vi "Acceleration.vi"() -> ()   [LabVIEW 2021]
uses:
  <vilib>/Instr/_visa.llb/VISA Configure Serial Port (Instr).vi
panel:
  out "AccelZ Chart":dbl(graph)
  out "AccelZ":dbl
  out "AccelY Chart":dbl(graph)
  out "AccelY":dbl
  out "AccelX Chart":dbl(graph)
  out "AccelX":dbl
  in  "stop":bool
  out "read buffer":string
  in  "baud rate (9600)":u32=9600
  in  "VISA resource name":refnum<visa-resource-name>
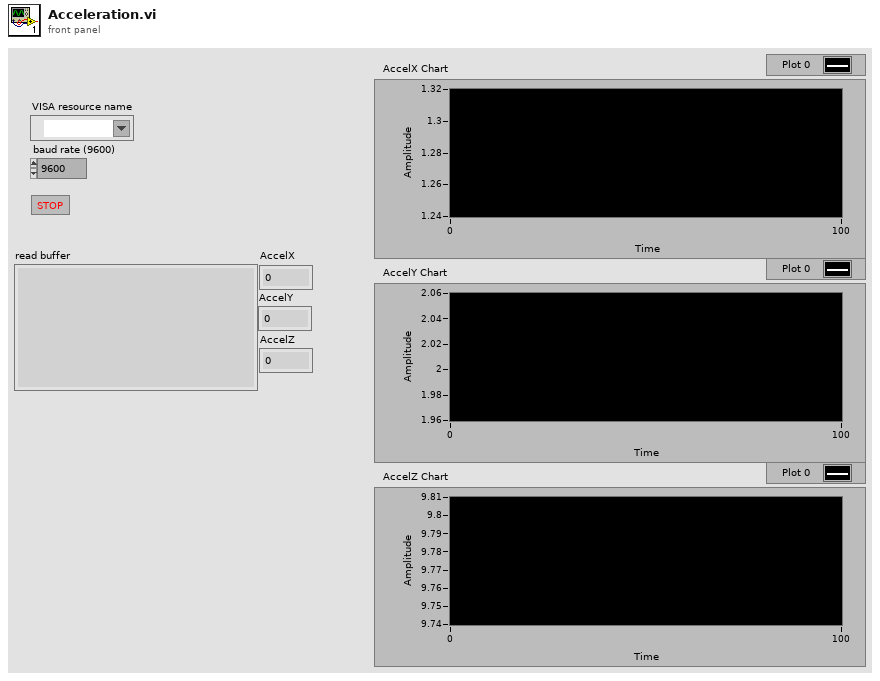
[diagram p1: front panel]
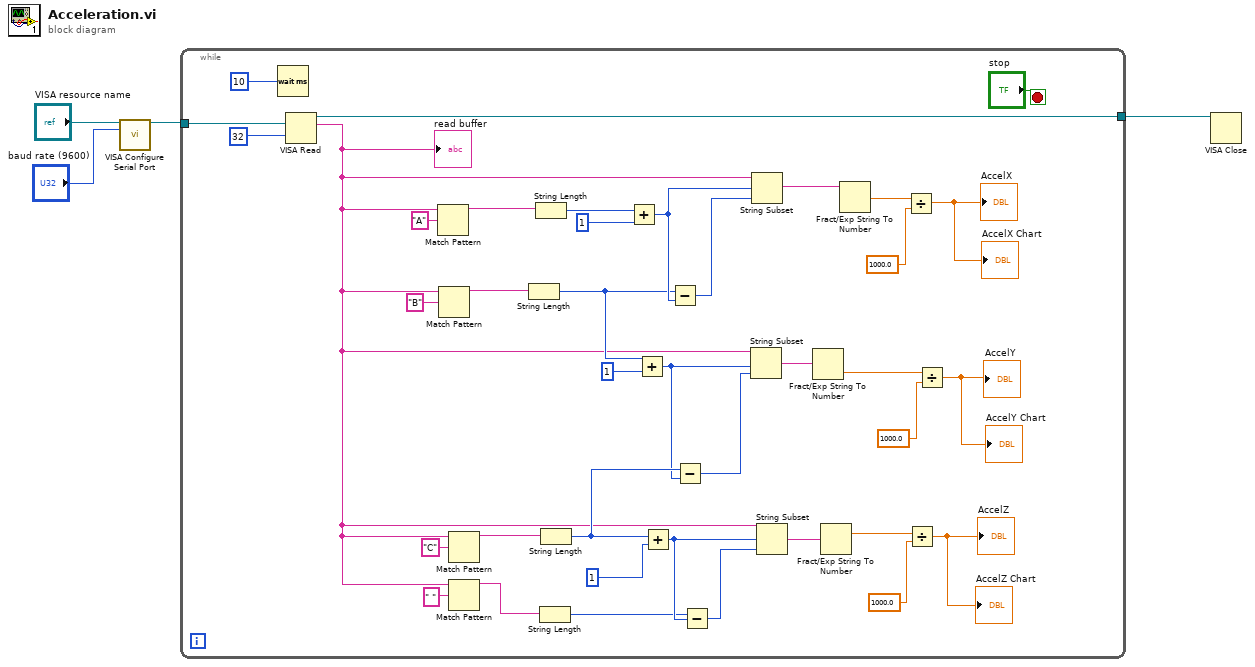
[diagram p0: block diagram]
diagram:
  n1 = call-poly "VISA Configure Serial Port"("VISA resource name"="VISA resource name", "baud rate (9600)"="baud rate (9600)") -> ("VISA resource name out"=w2:refnum<visa-resource-name>)  [unwired: 12 in, 1 out]
  n2 = while {
    tunnel: w2 -> [w43]
    tunnel: [w40] -> w1
    stop <- "stop" stop-if-true
    n3 = Wait (ms)(milliseconds to wait=u32 10) -> ()  [unwired: 1 out]
    n4 = VISA Read(VISA resource name=w43, byte count=u32 32) -> (VISA resource name out=w40:refnum<visa-resource-name>, read buffer=w15:string)  [unwired: 1 in, 2 out]
    "read buffer" <- w15
    n5 = Match Pattern(string=w15, regular expression="A") -> (before substring=w24:string)  [unwired: 1 in, 3 out]
    n6 = Match Pattern(string=w15, regular expression="B") -> (before substring=w34:string)  [unwired: 1 in, 3 out]
    n7 = Match Pattern(string=w15, regular expression="C") -> (before substring=w31:string)  [unwired: 1 in, 3 out]
    n8 = Match Pattern(string=w15, regular expression=" ") -> (before substring=w20:string)  [unwired: 1 in, 3 out]
    n9 = String Length(string=w34) -> (length=w27:i32)
    n10 = String Length(string=w24) -> (length=w36:i32)
    n11 = String Length(string=w20) -> (length=w14:i32)
    n12 = String Length(string=w31) -> (length=w26:i32)
    n13 = Add(x=w36, y=1) -> (x+y=w33:i32)
    n14 = Add(x=w27, y=1) -> (x+y=w25:i32)
    n15 = Add(x=w26, y=1) -> (x+y=w22:i32)
    n16 = Subtract(x=w27, y=w33) -> (x-y=w19:i32)
    n17 = Subtract(x=w26, y=w25) -> (x-y=w28:i32)
    n18 = Subtract(x=w14, y=w22) -> (x-y=w23:i32)
    n19 = String Subset(string=w15, offset (0)=w25, length (rest)=w28) -> (substring=w17:string)
    n20 = String Subset(string=w15, offset (0)=w33, length (rest)=w19) -> (substring=w18:string)
    n21 = String Subset(string=w15, offset (0)=w22, length (rest)=w23) -> (substring=w16:string)
    n22 = Fract/Exp String To Number(string=w17) -> (number=w9:dbl)  [unwired: 3 in, 1 out]
    n23 = Fract/Exp String To Number(string=w16) -> (number=w5:dbl)  [unwired: 3 in, 1 out]
    n24 = Fract/Exp String To Number(string=w18) -> (number=w6:dbl)  [unwired: 3 in, 1 out]
    n25 = Divide(x=w6, y=1000.0) -> (x/y=→"AccelX" →"AccelX Chart":dbl)
    n26 = Divide(x=w5, y=1000.0) -> (x/y=→"AccelZ" →"AccelZ Chart":dbl)
    n27 = Divide(x=w9, y=1000.0) -> (x/y=→"AccelY" →"AccelY Chart":dbl)
  }
  n28 = VISA Close(VISA resource name=w1) -> ()  [unwired: 1 in, 1 out]
